vi "main_jgxu_single2450.vi"() -> ()   [LabVIEW 2012]
panel:
  in  "Quit":bool
  out "XY Graph":cluster{dbl[], dbl[]}[](graph)
  in  "Mode":enum32{"Main Panel", "0254 Initialize"}(tab)
  out "Boolean 2":bool
  in  "Start_2400":bool
  out "Time (s)":dbl
  in  "Delay (ms)":u32=1000
  in  "Target (V)":dbl=0.01
  in  "Step (V)":dbl=0.001
  in  "Stop":bool
  in  "file path (use dialog)":path=path "D:/TD/20171028/mOs2/test.txt"
  in  "Ch1 Set":dbl
  out "Ch1 PV":dbl
  in  "Set Ch1":bool
  out "Boolean":bool
  out "SV_CH1":dbl
  in  "Ch2 Set Set":dbl
  out "SV_CH2":dbl
  out "Ch2 PV":dbl
  in  "Set Ch2":bool
  in  "VISA 2400":refnum<visa-resource-name>
  in  "VISA 0254":refnum<visa-resource-name>
  in  "Gas Flow Enable":bool
  in  "Initialization":bool
  out "Initiliazation Started":bool
  # "sccm"
  # "sccm"
  # "sccm"
  # "sccm"
  # "sccm"
  # "sccm"
  # "Please Wait  ~ 25 s"
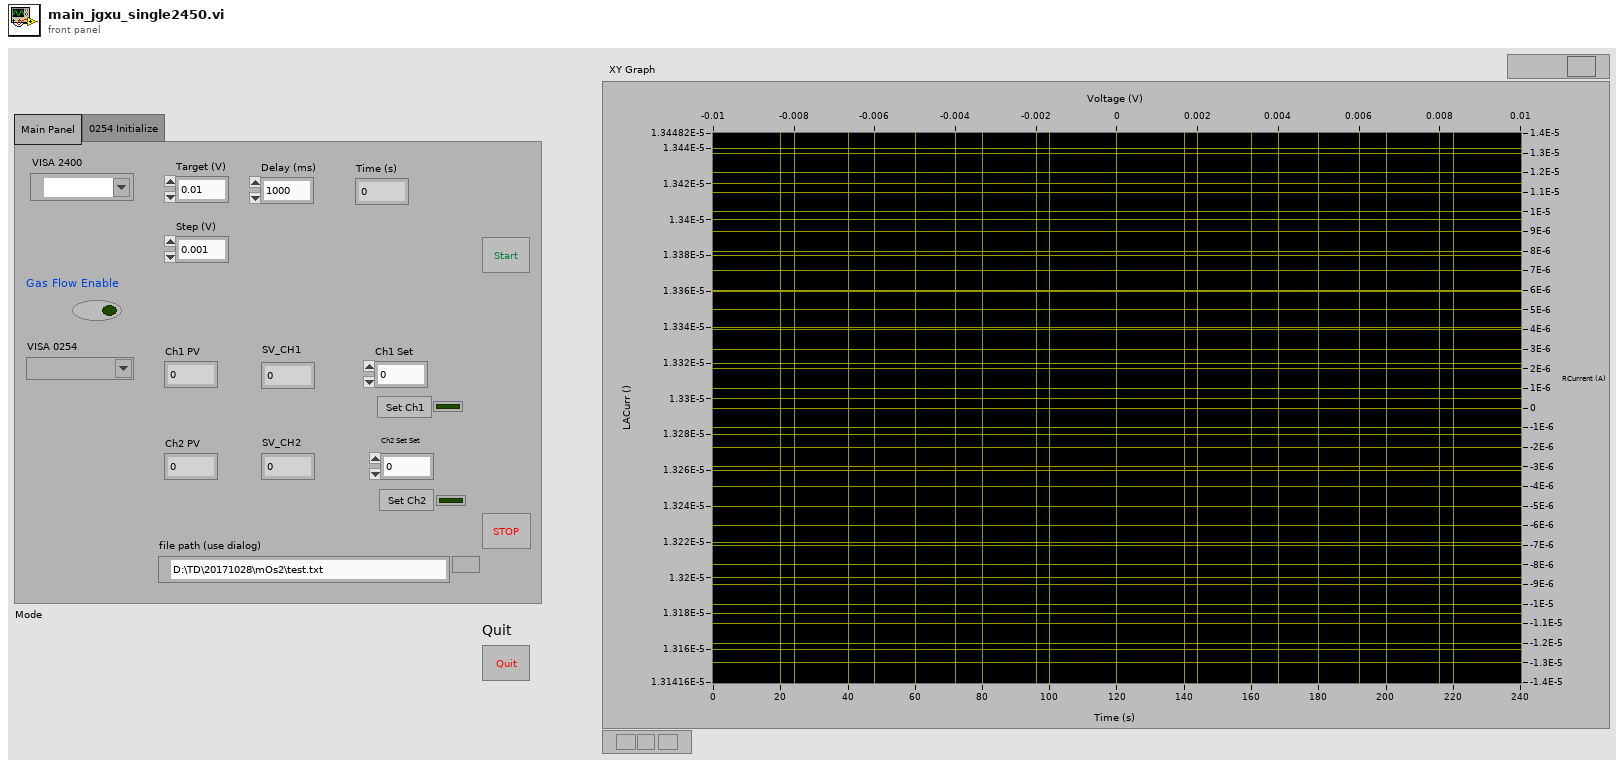
[diagram p1: front panel]
types:
  T1 = enum16{"open", "replace", "create", "open or create", "replace or create", "replace or create with confirmation"}
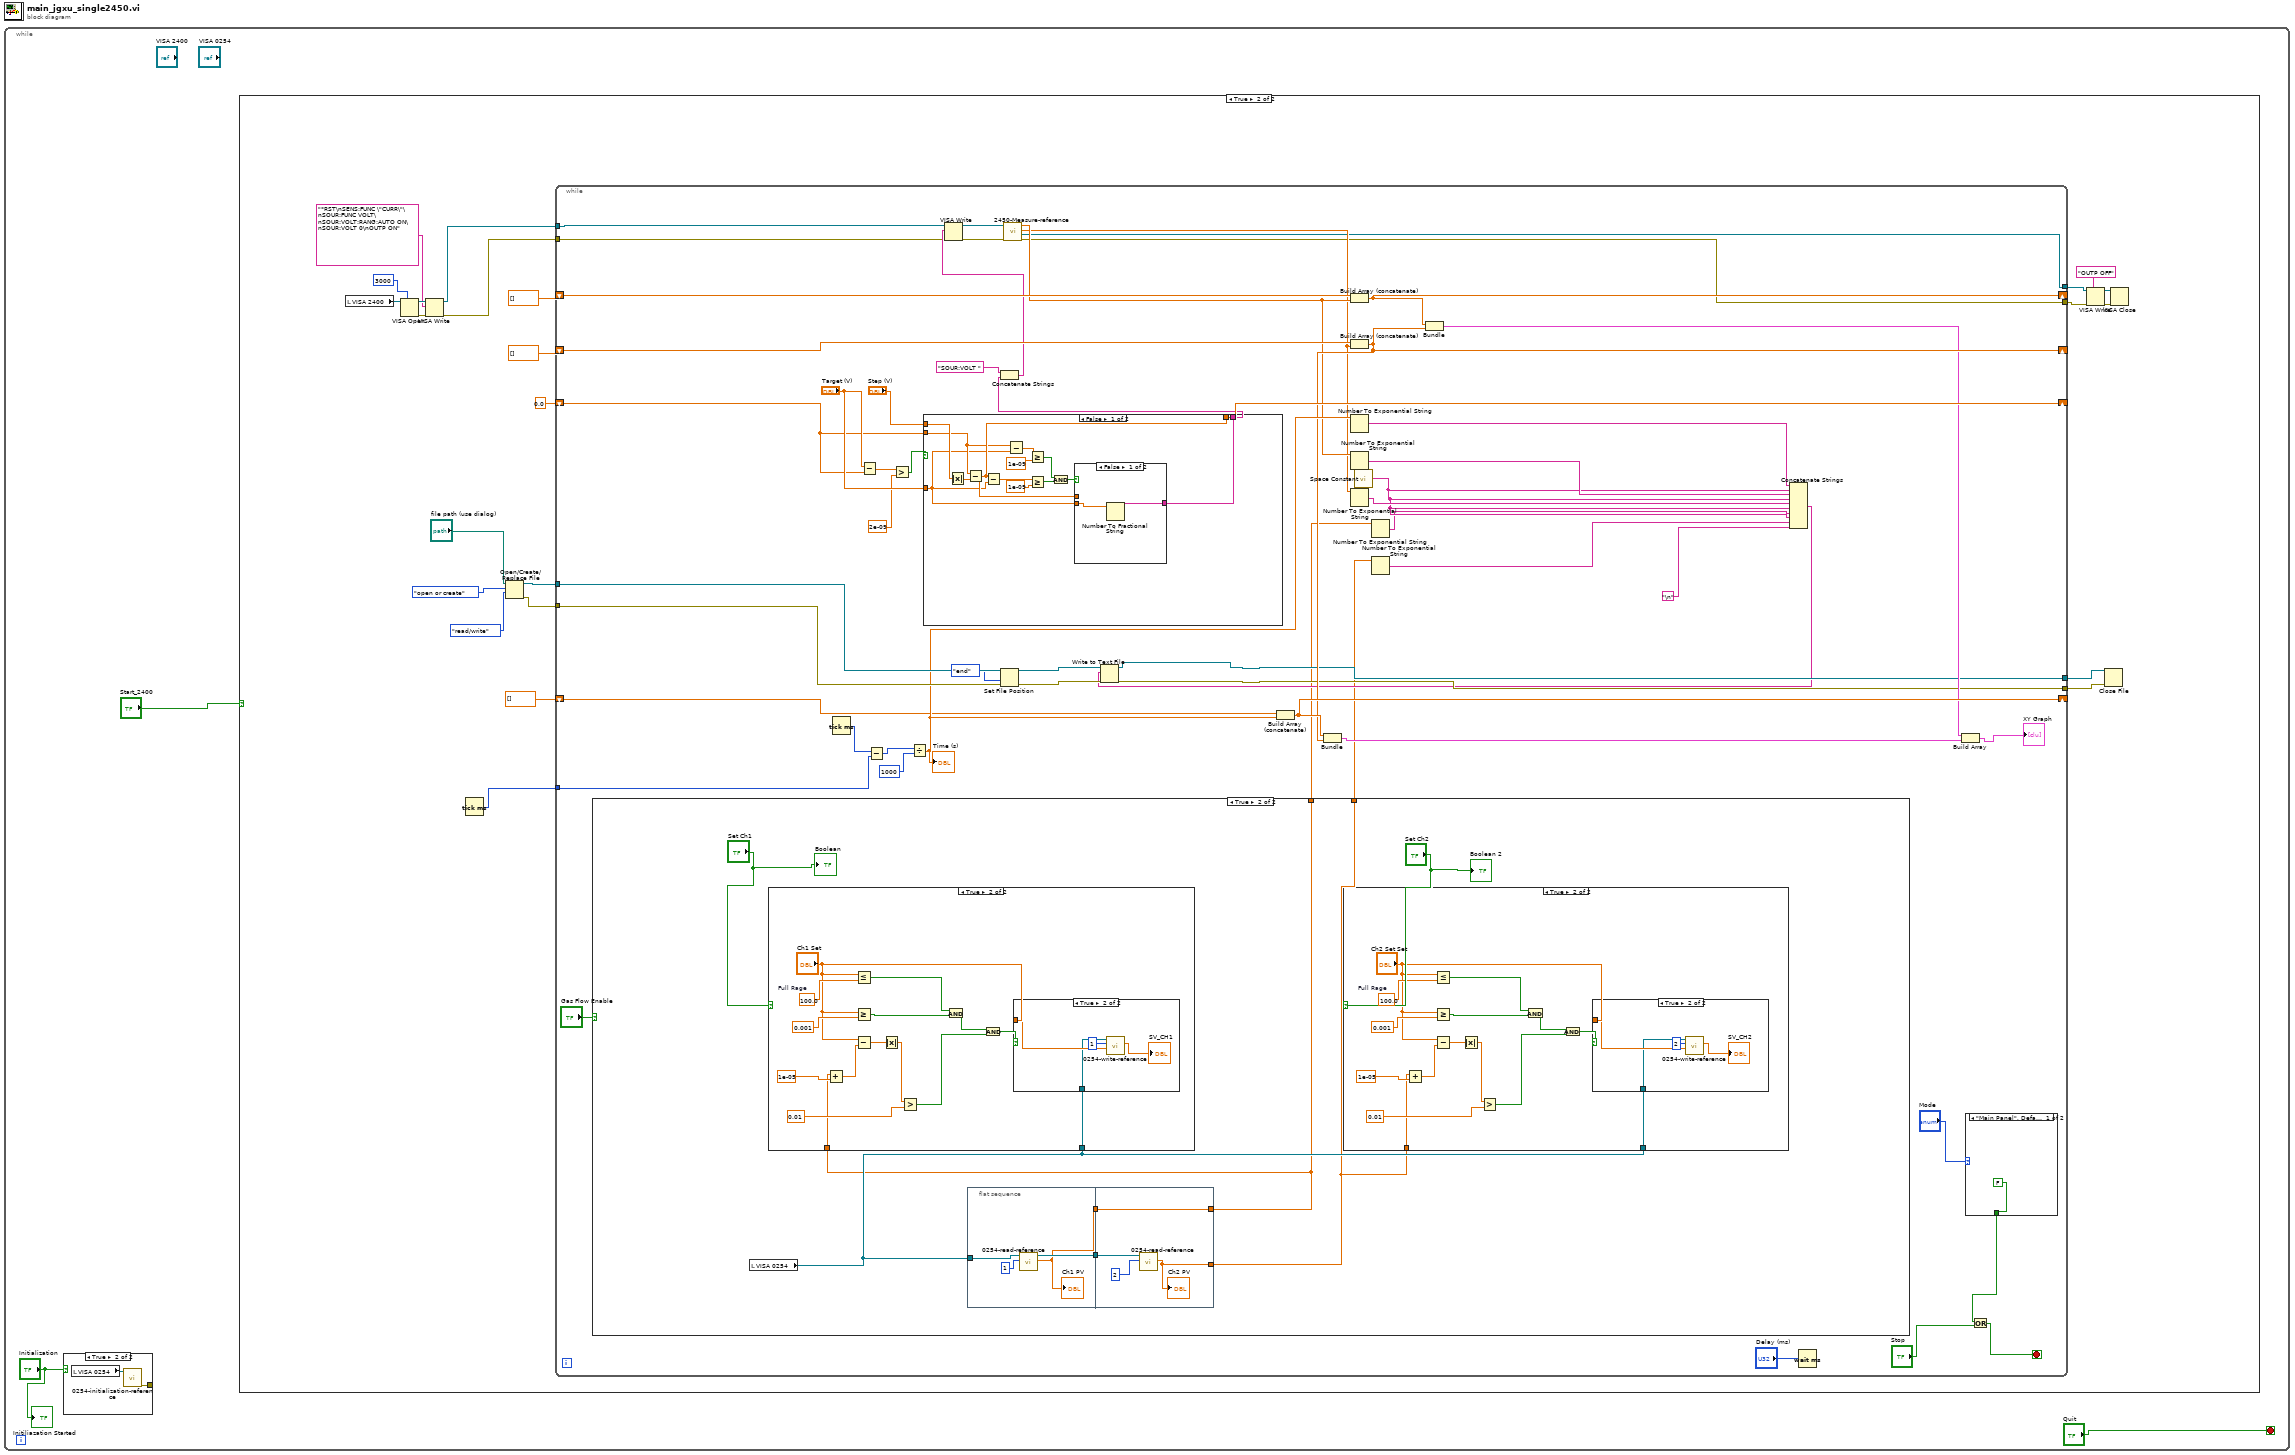
[diagram p0: block diagram]
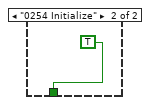
[diagram p3: hidden frame]
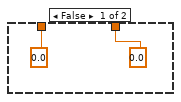
[diagram p4: hidden frame]
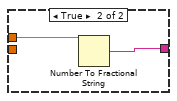
[diagram p9: hidden frame]
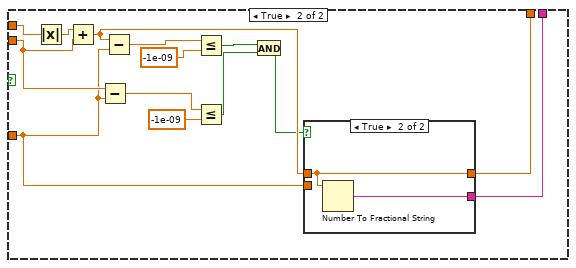
[diagram p10: hidden frame]
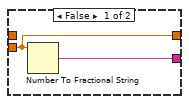
[diagram p11: hidden frame]
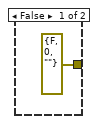
[diagram p12: hidden frame]
diagram:
  n1 = while {
    stop <- "Quit" stop-if-true
    n2 = case shown="True" "Initialization" {
      tunnel: [errorcluster {"status"=FALSE, "code"=0, "source"=""} ("error out") w176] -> _
      frame False {
      }
      frame True {
        n3 = local read "VISA 0254"() -> (w177:refnum<visa-resource-name>)
        n4 = call "0254-initialization-reference.vi"("0254-VISA"=w177) -> ("error out"=w176:errorcluster)  [unwired: 8 in, 2 out]
      }
    }
    n5 = case shown="True" "Start_2400" {
      frame False {
      }
      frame True {
        n6 = local read "VISA 2400"() -> (w13:refnum<visa-resource-name>)
        n7 = VISA Open(timeout (0)=3000 ("timeout ms (488.2 global)"), VISA resource name=w13) -> (VISA resource name=w16:refnum<visa-resource-name>, error out=w15:errorcluster)  [unwired: 3 in]
        n8 = VISA Write(VISA resource name=w16, write buffer="*RST\nSENS:FUNC \"CURR\"\nSOUR:FUNC VOLT\nSOUR:VOLT:RANG:AUTO ON\nSOUR:VOLT 0\nOUTP ON" ("data"), error in (no error)=w15) -> (VISA resource name out=w10:refnum<visa-resource-name>, error out=w11:errorcluster)  [unwired: 1 out]
        n9 = Tick Count (ms)() -> (millisecond timer value=w18:u32)
        n10 = Open/Create/Replace File(file path (use dialog)="file path (use dialog)", operation (0:open)=T1."open or create", access (0:read/write)=enum16{"read/write", "read-only", "write-only"}."read/write") -> (refnum out=w23:refnum<file>, error out=w22:errorcluster)  [unwired: 1 in, 3 out]
        n11 = while {
          shift-right: [w69] -> _
          shift-left: 0.0 ("Target (V)") -> [w65]
          shift-right: [w78] -> _
          shift-left: dbl[] [] -> [w81]
          shift-right: [w52] -> _
          shift-left: dbl[] [] -> [w80]
          tunnel: w23 -> [w75]
          tunnel: w22 -> [w74]
          tunnel: [w46] -> w21
          tunnel: [w47] -> w20
          tunnel: w10 -> [w61]
          tunnel: [w38] -> w6
          tunnel: [w37] -> w5
          tunnel: w11 -> [w51]
          tunnel: w18 -> [w59]
          shift-right: [w53] -> _
          shift-left: dbl[] [] -> [w54]
          stop <- w32 stop-if-true
          n12 = case shown="True" "Gas Flow Enable" {
            tunnel: [0.0 ("PV") w88] -> w44
            tunnel: [0.0 ("PV") w87] -> w43
            frame False {
            }
            frame True {
              n13 = local read "VISA 0254"() -> (w92:refnum<visa-resource-name>)
              n14 = case shown="True" "Set Ch1" {
                tunnel: w92 -> [_ w122]
                tunnel: w88 -> [_ w121]
                frame False {
                }
                frame True {
                  w125 = 100.0  # Full Rage
                  n15 = Add(x=w121, y=1e-05) -> (x+y=w134:dbl)
                  n16 = Less Or Equal?(x="Ch1 Set", y=w125) -> (x <= y?=w127:bool)
                  n17 = Greater Or Equal?(x="Ch1 Set", y=0.001) -> (x >= y?=w128:bool)
                  n18 = Subtract(x="Ch1 Set", y=w134) -> (x-y=w129:dbl)
                  n19 = Absolute Value(x=w129) -> (abs(x)=w130:dbl)
                  n20 = Greater?(x=w130, y=0.01) -> (0:w133:bool)
                  n21 = And(x=w127, y=w128) -> (x .and. y?=w132:bool)
                  n22 = And(x=w132, y=w133) -> (x .and. y?=w124:bool)
                  n23 = case shown="True" w124 {
                    tunnel: "Ch1 Set" -> [_ w139]
                    tunnel: w122 -> [_ w137]
                    frame False {
                    }
                    frame True {
                      n24 = call "0254-write-reference.vi"("SV"=w139, "Channel Selection"=1, "VISA Refnum in"=w137) -> ("SV_CH1"=→"SV_CH1":dbl)  [unwired: 6 in, 2 out]
                    }
                  }
                }
              }
              n25 = flat-sequence {
                tunnel: w92 -> [w96]
                tunnel: [w95] -> w90
                tunnel: [w94] -> w89
                tunnel: w90 -> [w100]
                tunnel: w89 -> [w99]
                tunnel: [w99] -> w88
                tunnel: [w98] -> w87
                frame #0 {
                  n26 = call "0254-read-reference.vi"("Channel Selction"=1, "VISA Refnum in"=w96) -> ("PV"=w94:dbl, "VISA Refnum out"=w95:refnum<visa-resource-name>)  [unwired: 7 in, 1 out]
                  "Ch1 PV" <- w94
                }
                frame #1 {
                  n27 = call "0254-read-reference.vi"("Channel Selction"=2 ("Channel Selction 2"), "VISA Refnum in"=w100) -> ("PV"=w98:dbl)  [unwired: 7 in, 2 out]
                  "Ch2 PV" <- w98
                }
              }
              n28 = case shown="True" "Set Ch2" {
                tunnel: w92 -> [_ w103]
                tunnel: w87 -> [_ w102]
                frame False {
                }
                frame True {
                  w106 = 100.0  # Full Rage
                  n29 = Add(x=w102, y=1e-05) -> (x+y=w115:dbl)
                  n30 = Less Or Equal?(x="Ch2 Set Set", y=w106) -> (x <= y?=w108:bool)
                  n31 = Greater Or Equal?(x="Ch2 Set Set", y=0.001) -> (x >= y?=w109:bool)
                  n32 = Subtract(x="Ch2 Set Set", y=w115) -> (x-y=w110:dbl)
                  n33 = Absolute Value(x=w110) -> (abs(x)=w111:dbl)
                  n34 = Greater?(x=w111, y=0.01) -> (0:w114:bool)
                  n35 = And(x=w108, y=w109) -> (x .and. y?=w113:bool)
                  n36 = And(x=w113, y=w114) -> (x .and. y?=w105:bool)
                  n37 = case shown="True" w105 {
                    tunnel: "Ch2 Set Set" -> [_ w120]
                    tunnel: w103 -> [_ w118]
                    frame False {
                    }
                    frame True {
                      n38 = call "0254-write-reference.vi"("SV"=w120, "Channel Selection"=2, "VISA Refnum in"=w118) -> ("SV_CH1"=→"SV_CH2":dbl)  [unwired: 6 in, 2 out]
                    }
                  }
                }
              }
              "Boolean" <- "Set Ch1"
              "Boolean 2" <- "Set Ch2"
            }
          }
          n39 = Tick Count (ms)() -> (millisecond timer value=w58:u32)
          n40 = Subtract(x="Target (V)", y=w65) -> (x-y=w64:dbl)
          n41 = Subtract(x=w58, y=w59) -> (x-y=w57:u32)
          n42 = Greater?(x=w64, y=2e-09) -> (0:w68:bool)
          n43 = Divide(x=w57, y=u32 1000) -> (x/y=w55:dbl)
          "Time (s)" <- w55
          n44 = case shown="False" w68 {
            tunnel: "Step (V)" -> [w152 w170]
            tunnel: w65 -> [w147 w165]
            tunnel: "Target (V)" -> [w146 w164]
            tunnel: [w149 w167] -> w69
            tunnel: [w148 w166] -> w67
            frame False {
              n45 = Absolute Value(x=w152) -> (abs(x)=w151:dbl)
              n46 = Subtract(x=w147, y=w151) -> (x-y=w149:dbl)
              n47 = Subtract(x=w149, y=w146) -> (x-y=w141:dbl)
              n48 = Subtract(x=w147, y=w146) -> (x-y=w140:dbl)
              n49 = Greater Or Equal?(x=w140, y=1e-09) -> (x >= y?=w144:bool)
              n50 = Greater Or Equal?(x=w141, y=1e-09) -> (x >= y?=w143:bool)
              n51 = And(x=w144, y=w143) -> (x .and. y?=w142:bool)
              n52 = case shown="False" w142 {
                tunnel: w149 -> [_ w156]
                tunnel: [w153 w155] -> w148
                tunnel: w146 -> [w154 _]
                frame False {
                  n53 = Number To Fractional String(number=w154) -> (F-format string=w153:string)  [unwired: 3 in]
                }
                frame True {
                  n54 = Number To Fractional String(number=w156) -> (F-format string=w155:string)  [unwired: 3 in]
                }
              }
            }
            frame True {
              n55 = Absolute Value(x=w170) -> (abs(x)=w169:dbl)
              n56 = Add(x=w169, y=w165) -> (x+y=w168:dbl)
              n57 = Subtract(x=w165, y=w164) -> (x-y=w159:dbl)
              n58 = Subtract(x=w168, y=w164) -> (x-y=w162:dbl)
              n59 = Less Or Equal?(x=w162, y=-1e-09) -> (x <= y?=w160:bool)
              n60 = Less Or Equal?(x=w159, y=-1e-09) -> (x <= y?=w157:bool)
              n61 = And(x=w160, y=w157) -> (x .and. y?=w163:bool)
              n62 = case shown="True" w163 {
                tunnel: w168 -> [_ w173]
                tunnel: [w172 w174] -> w166
                tunnel: w164 -> [w171 _]
                tunnel: [w171 w173] -> w167
                frame False {
                  n63 = Number To Fractional String(number=w171) -> (F-format string=w172:string)  [unwired: 3 in]
                }
                frame True {
                  n64 = Number To Fractional String(number=w173) -> (F-format string=w174:string)  [unwired: 3 in]
                }
              }
            }
          }
          n65 = Concatenate Strings("SOUR:VOLT " ("string"), w67) -> (w62:string)
          n66 = VISA Write(VISA resource name=w61, write buffer=w62, error in (no error)=w51) -> (VISA resource name out=w42:refnum<visa-resource-name>, error out=w41:errorcluster)  [unwired: 1 out]
          n67 = Set File Position(refnum=w75, from (0:start)=enum16{"start", "end", "current"}."end", error in=w74) -> (refnum out=w73:refnum<file>, error out=w72:errorcluster)  [unwired: 1 out]
          n68 = call "2450-Measure-reference.vi"("error in (no error)"=w41, "VISA Refnum in"=w42) -> ("error out"=w37:errorcluster, "VISA resource name out"=w38:refnum<visa-resource-name>, "Current Output"=w39:dbl, "Voltage Output"=w40:dbl)  [unwired: 6 in]
          n69 = Build Array (concatenate)(w54, w55) -> (w53:dbl[])
          n70 = Build Array (concatenate)(w81, w40) -> (w78:dbl[])
          n71 = Build Array (concatenate)(w80, w39) -> (w52:dbl[])
          n72 = Bundle(w53, w52) -> (w49:cluster{dbl[], dbl[]})  [unwired: 1 in]
          n73 = Number To Exponential String(number=w55) -> (E-format string=w56:string)  [unwired: 3 in]
          n74 = Number To Exponential String(number=w40) -> (E-format string=w76:string)  [unwired: 3 in]
          n75 = Number To Exponential String(number=w39) -> (E-format string=w77:string)  [unwired: 3 in]
          n76 = call <vilib>:"Space Constant.vi"() -> ("String"=w31:string)
          n77 = Number To Exponential String(number=w44) -> (E-format string=w30:string)  [unwired: 3 in]
          n78 = Number To Exponential String(number=w43) -> (E-format string=w29:string)  [unwired: 3 in]
          n79 = Bundle(w78, w52) -> (w50:cluster{dbl[], dbl[]})  [unwired: 1 in]
          n80 = Concatenate Strings(w56, w31, w76, w31, w77, w31, w30, w31, w29, "\n") -> (w45:string)
          n81 = Write to Text File(file (use dialog)=w73, text=w45, error in=w72) -> (refnum out=w47:refnum<file>, error out=w46:errorcluster)  [unwired: 1 in, 1 out]
          n82 = Wait (ms)(milliseconds to wait="Delay (ms)") -> ()  [unwired: 1 out]
          n83 = Build Array(w50, w49) -> (→"XY Graph":cluster{dbl[], dbl[]}[])
          n84 = case shown="\"Main Panel\", Default" "Mode" {
            tunnel: [FALSE TRUE] -> w34
            frame "Main Panel", Default {
            }
            frame "0254 Initialize" {
            }
          }
          n85 = Or(x=w34, y="Stop") -> (x .or. y?=w32:bool)
        }
        n86 = VISA Write(VISA resource name=w6, write buffer="OUTP OFF" ("data"), error in (no error)=w5) -> (VISA resource name out=w8:refnum<visa-resource-name>, error out=w7:errorcluster)  [unwired: 1 out]
        n87 = Close File(refnum=w20, error in=w21) -> ()  [unwired: 2 out]
        n88 = VISA Close(VISA resource name=w8, error in (no error)=w7) -> ()  [unwired: 1 out]
      }
    }
    "Initiliazation Started" <- "Initialization"
  }
